vi "Rinocloud_JSON_encoder.vi"(8 "self ID":string="name", 9 "parent ID":string="name", 10 "Extra metadata array":T1(array[cluster])=[{"Attribute"="", "Value"="", "Data type"=enum."<null>"}], 11 "Metadata":T2) -> (3 "JSON payload":string)   [LabVIEW 2013]
uses:
  i3 JSON/JSON Generation/Create Value Files/Create Value - Object.vi
  i3 JSON/JSON Generation/Add Object Parameter Files/Add Object Parameter - String.vi
  i3 JSON/JSON Generation/Add Object Parameter Files/Add Object Parameter - 1D Array String.vi
  i3 JSON/JSON Generation/Add Object Parameter Files/Add Object Parameter - Numeric.vi
  i3 JSON/JSON Generation/Add Object Parameter Files/Add Object Parameter - 1D Array Double.vi
  i3 JSON/JSON Generation/Add Object Parameter Files/Add Object Parameter - Data JSON string.vi
  i3 JSON/i3-json.lvlib
panel:
  out "error out":errorcluster
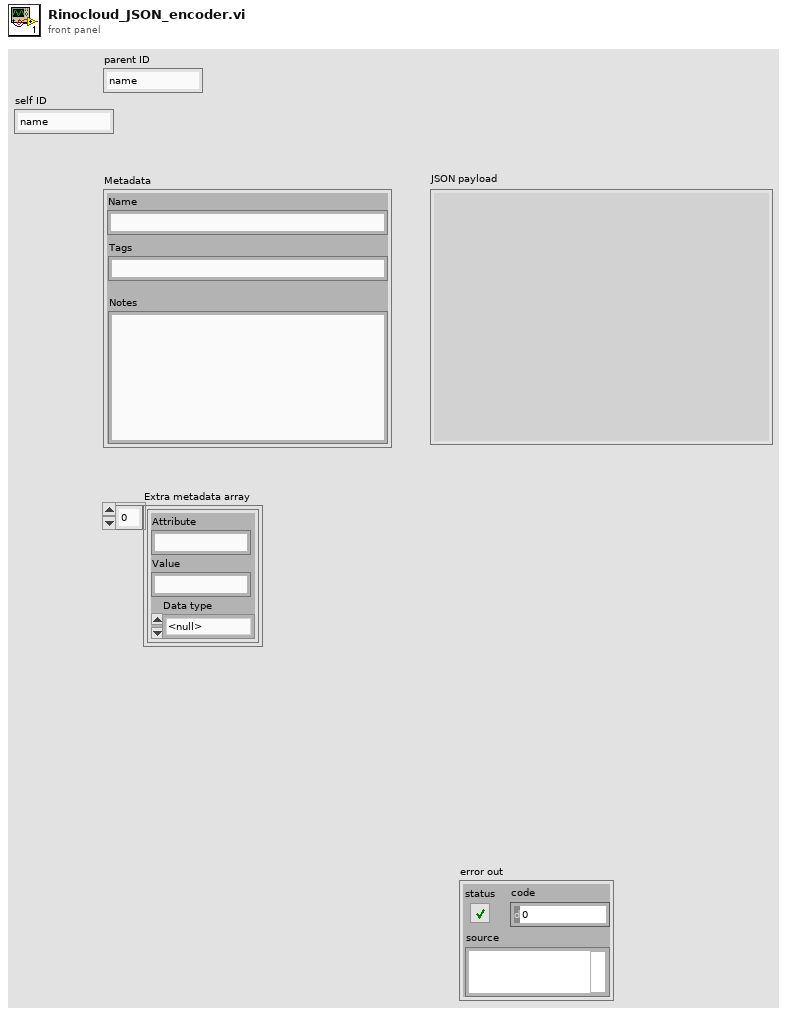
[diagram p1: front panel]
types:
  T1 = cluster{"Attribute":string, "Value":string, "Data type":enum16{"Numeric", "String", "1D array of strings", "1D array of doubles", "Data JSON string", "<null>"}}[]
  T2 = cluster{"Name":string, "Notes":string, "Tags":string}
  T3 = enum16{"Numeric", "String", "1D array of strings", "1D array of doubles", "Data JSON string", "<null>"}
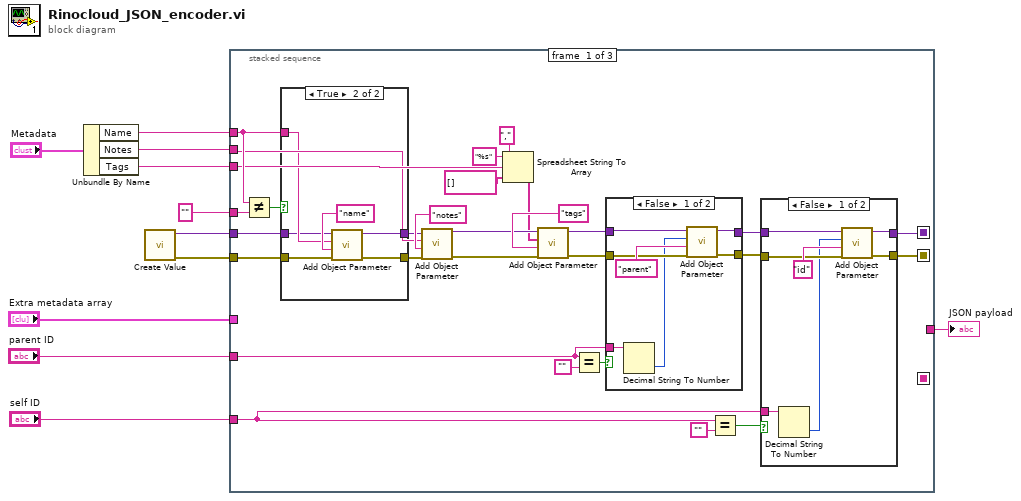
[diagram p0: block diagram]
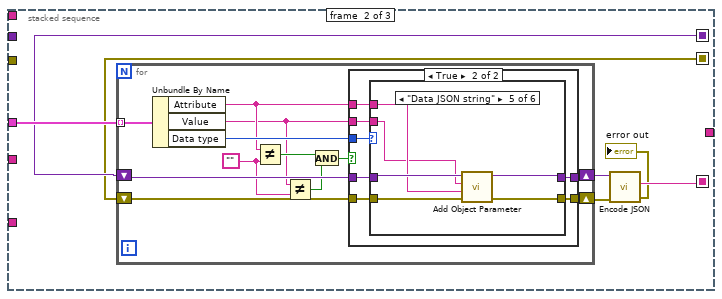
[diagram p5: hidden frame]
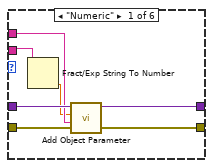
[diagram p7: hidden frame]
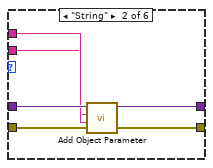
[diagram p8: hidden frame]
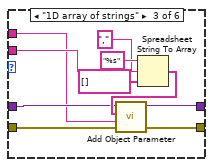
[diagram p9: hidden frame]
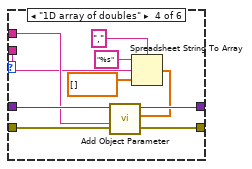
[diagram p10: hidden frame]
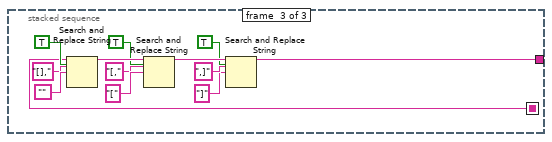
[diagram p12: hidden frame]
diagram:
  n1 = Unbundle By Name("Metadata") -> ("Name"=w7:string, "Notes"=w5:string, "Tags"=w6:string)
  n2 = call-poly "Create Value.vi"() -> ("error out"=w3:errorcluster, "JSON Tree"=w10:variant)  [unwired: 10 in]
  n3 = stacked-sequence {
    seq-local: [_ w72 _] -> [_ _ w136]
    seq-local: [w16 _ _] -> [_ w68 _]
    seq-local: [w15 _ _] -> [_ w67 _]
    tunnel: w7 -> [w38 _ _]
    tunnel: w5 -> [w27 _ _]
    tunnel: w6 -> [w30 _ _]
    tunnel: w10 -> [w39 _ _]
    tunnel: "" ("y") -> [w37 _ _]
    tunnel: "Extra metadata array" -> [_ w73 _]
    tunnel: [_ _ w137] -> w9
    tunnel: w3 -> [w36 _ _]
    tunnel: "parent ID" -> [w19 _ _]
    tunnel: "self ID" -> [w12 _ _]
    frame #0 {
      n4 = Not Equal?(x=w38, y=w37) -> (x != y?=w40:bool)
      n5 = case shown="True" w40 {
        tunnel: w39 -> [w60 w64]
        tunnel: w38 -> [_ w65]
        tunnel: [w60 w63] -> w29
        tunnel: w36 -> [w59 w62]
        tunnel: [w59 w61] -> w28
        frame False {
        }
        frame True {
          n6 = call-poly "Add Object Parameter.vi"("error in (no error)"=w62, "Name"="name", "String"=w65, "JSON Tree in (JSON Object)"=w64) -> ("error out"=w61:errorcluster, "JSON Tree out (JSON Object)"=w63:variant)  [unwired: 6 in]
        }
      }
      n7 = call-poly "Add Object Parameter.vi"("error in (no error)"=w28, "Name"="notes", "String"=w27, "JSON Tree in (JSON Object)"=w29) -> ("error out"=w25:errorcluster, "JSON Tree out (JSON Object)"=w26:variant)  [unwired: 6 in]
      n8 = Spreadsheet String To Array(delimiter (Tab)=",", format string="%s", spreadsheet string=w30, array type (2D Dbl)=string[] [] ("Array")) -> (array=w24:string[])
      n9 = call-poly "Add Object Parameter.vi"("error in (no error)"=w25, "Name"="tags", "1D String"=w24, "JSON Tree in (JSON Object)"=w26) -> ("error out"=w21:errorcluster, "JSON Tree out (JSON Object)"=w22:variant)  [unwired: 6 in]
      n10 = Equal?(x=w19, y="") -> (x = y?=w20:bool)
      n11 = case shown="False" w20 {
        tunnel: w22 -> [w54 w58]
        tunnel: [w55 w58] -> w18
        tunnel: [w56 w57] -> w17
        tunnel: w21 -> [w52 w57]
        tunnel: w19 -> [w51 _]
        frame False {
          n12 = Decimal String To Number(string=w51) -> (number=w50:i32)  [unwired: 2 in, 1 out]
          n13 = call-poly "Add Object Parameter.vi"("error in (no error)"=w52, "Name"="parent", "Numeric"=w50, "JSON Tree in (JSON Object)"=w54) -> ("error out"=w56:errorcluster, "JSON Tree out (JSON Object)"=w55:variant)  [unwired: 6 in]
        }
        frame True {
        }
      }
      n14 = Equal?(x=w12, y="") -> (x = y?=w13:bool)
      n15 = case shown="False" w13 {
        tunnel: w18 -> [w45 w49]
        tunnel: [w46 w49] -> w16
        tunnel: [w47 w48] -> w15
        tunnel: w17 -> [w43 w48]
        tunnel: w12 -> [w42 _]
        frame False {
          n16 = Decimal String To Number(string=w42) -> (number=w41:i32)  [unwired: 2 in, 1 out]
          n17 = call-poly "Add Object Parameter.vi"("error in (no error)"=w43, "Name"="id", "Numeric"=w41, "JSON Tree in (JSON Object)"=w45) -> ("error out"=w47:errorcluster, "JSON Tree out (JSON Object)"=w46:variant)  [unwired: 6 in]
        }
        frame True {
        }
      }
    }
    frame #1 {
      n18 = for {
        tunnel: w73 -> [w85] mode=indexing
        shift-right: [w80] -> w71
        shift-left: w68 -> [w81]
        shift-right: [w82] -> w69
        shift-left: w67 -> [w83]
        w75 = ""
        n19 = Unbundle By Name(w85) -> ("Attribute"=w79:string, "Value"=w74:string, "Data type"=w84:T3)
        n20 = Not Equal?(x=w79, y=w75) -> (x != y?=w77:bool)
        n21 = Not Equal?(x=w74, y=w75) -> (x != y?=w76:bool)
        n22 = And(x=w77, y=w76) -> (x .and. y?=w78:bool)
        n23 = case shown="True" w78 {
          tunnel: w84 -> [_ w94]
          tunnel: w83 -> [w86 w93]
          tunnel: [w86 w92] -> w82
          tunnel: w81 -> [w87 w91]
          tunnel: [w87 w90] -> w80
          tunnel: w79 -> [_ w89]
          tunnel: w74 -> [_ w88]
          frame False {
          }
          frame True {
            n24 = case shown="\"Data JSON string\"" w94 {
              tunnel: w93 -> [w101 w104 w112 w125 w133 w134]
              tunnel: [w100 w105 w108 w123 w132 w134] -> w92
              tunnel: w91 -> [w99 w107 w113 w126 w131 w135]
              tunnel: [w98 w106 w109 w124 w130 w135] -> w90
              tunnel: w89 -> [w97 w103 w110 w122 w129 _]
              tunnel: w88 -> [w95 w102 w111 w121 w128 _]
              frame "Numeric" {
                n25 = Fract/Exp String To Number(string=w95) -> (number=w96:dbl)  [unwired: 3 in, 1 out]
                n26 = call-poly "Add Object Parameter.vi"("error in (no error)"=w101, "Name"=w97, "Numeric"=w96, "JSON Tree in (JSON Object)"=w99) -> ("error out"=w100:errorcluster, "JSON Tree out (JSON Object)"=w98:variant)  [unwired: 6 in]
              }
              frame "String" {
                n27 = call-poly "Add Object Parameter.vi"("error in (no error)"=w104, "Name"=w103, "String"=w102, "JSON Tree in (JSON Object)"=w107) -> ("error out"=w105:errorcluster, "JSON Tree out (JSON Object)"=w106:variant)  [unwired: 6 in]
              }
              frame "1D array of strings" {
                n28 = Spreadsheet String To Array(delimiter (Tab)=",", format string="%s", spreadsheet string=w111, array type (2D Dbl)=string[] [] ("Array")) -> (array=w115:string[])
                n29 = call-poly "Add Object Parameter.vi"("error in (no error)"=w112, "Name"=w110, "1D String"=w115, "JSON Tree in (JSON Object)"=w113) -> ("error out"=w108:errorcluster, "JSON Tree out (JSON Object)"=w109:variant)  [unwired: 6 in]
              }
              frame "1D array of doubles" {
                n30 = Spreadsheet String To Array(delimiter (Tab)=",", format string="%s", spreadsheet string=w121, array type (2D Dbl)=dbl[] []) -> (array=w118:dbl[])
                n31 = call-poly "Add Object Parameter.vi"("error in (no error)"=w125, "Name"=w122, "1D Double"=w118, "JSON Tree in (JSON Object)"=w126) -> ("error out"=w123:errorcluster, "JSON Tree out (JSON Object)"=w124:variant)  [unwired: 6 in]
              }
              frame "Data JSON string" {
                n32 = call-poly "Add Object Parameter.vi"("error in (no error)"=w133, "Name"=w129, "String"=w128, "JSON Tree in (JSON Object)"=w131) -> ("error out"=w132:errorcluster, "JSON Tree out (JSON Object)"=w130:variant)  [unwired: 6 in]
              }
              frame "<null>", Default {
              }
            }
          }
        }
      }
      n33 = call "Encode JSON.vi"("error in (no error)"=w69, "JSON Tree"=w71) -> ("error out"=→"error out":errorcluster, "String"=w72:string)  [unwired: 4 in]
    }
    frame #2 {
      n34 = Search and Replace String(replace all?=TRUE ("replace all? (F)"), input string=w136, search string="[],", replace string="") -> (result string=w143:string)  [unwired: 4 in, 3 out]
      n35 = Search and Replace String(replace all?=TRUE ("replace all? (F)"), input string=w143, search string="[,", replace string="[" ("search string")) -> (result string=w148:string)  [unwired: 4 in, 3 out]
      n36 = Search and Replace String(replace all?=TRUE ("replace all? (F)"), input string=w148, search string=",]", replace string="]" ("search string")) -> (result string=w137:string)  [unwired: 4 in, 3 out]
    }
  }
  "JSON payload" <- w9
